vi "DSF.Engine.Interface.Builder.Write.Response.vi"(6 "overwrite on timeout (T)":bool, 8 "error in (no error)":errorcluster, 9 "timeout in ms (0)":i32 format="%d ms", 10 "response":T1, 11 "Builder Interface in":refnum<class "DSF.Engine.Interface.Builder.lvclass">) -> (0 "error out":errorcluster, 1 "timed out?":bool, 3 "Builder Interface out":refnum<class "DSF.Engine.Interface.Builder.lvclass">)   [LabVIEW 2016, in "DSF.Engine.lvlib" / "DSF.Engine.Interface.Builder.lvclass"]
uses:
  DSF.Engine.Interface.Builder.lvclass
  C:/Git/Sourcetree/DSF/Source/Engine/Classes/Interface/DSF.Engine.Interface.lvclass
  DSF.Engine.Interface.Builder.Response Data.ctl
  DSF.Engine.Interface.Builder.Response.ctl
  DSF.Engine.Interface.lvclass/DSF.Engine.Interface.ctl
  DSF.Engine.Interface.lvclass
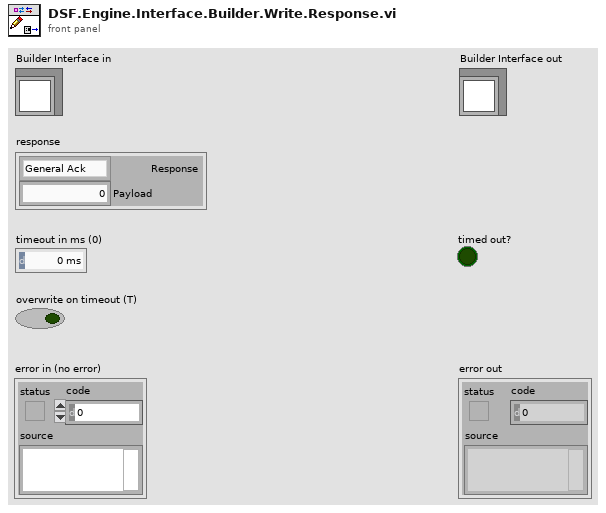
[diagram p1: front panel]
types:
  T1 = typedef "DSF.Engine.lvlib/DSF.Engine.Interface.Builder.lvclass/DSF.Engine.Interface.Builder.Response Data.ctl" = cluster{"Response":T2, "Payload":u64}
  T2 = typedef "DSF.Engine.lvlib/DSF.Engine.Interface.Builder.lvclass/DSF.Engine.Interface.Builder.Response.ctl" = enum8{"General Ack", "Shutdown Ack"}
  T3 = typedef "DSF.Engine.lvlib/DSF.Engine.Interface.lvclass/DSF.Engine.Interface.RT FIFO Ref.ctl" = refnum<k33>
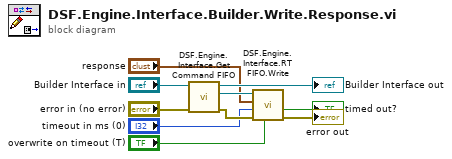
[diagram p0: block diagram]
diagram:
  n1 = call "DSF.Engine.Interface.Get Command FIFO.vi"("error in (no error)"="error in (no error)", "Interface in"="Builder Interface in") -> ("error out"=w9:errorcluster, "Command FIFO"=w10:T3, "Interface out"=→"Builder Interface out":refnum<class "DSF.Engine.Interface.Builder.lvclass">)  [unwired: 7 in]
  n2 = call "DSF.Engine.Interface.RT FIFO.Write.vi"("overwrite on timeout (T)"="overwrite on timeout (T)", "error in (no error)"=w9, "timeout in ms (0)"="timeout in ms (0)", "element"="response", "RT FIFO in"=w10) -> ("error out"=→"error out":errorcluster, "timed out?"=→"timed out?":bool)  [unwired: 4 in, 1 out]
